vi "Thorlabs Module.vi"(7 "Actions":T3(ring)=enum."Generate Scan Pattern", 8 "error in":errorcluster, 9 "Objective":u16(ring)=1 items=["5X LKM05", "10X LKM10", "20X LKM20", "10X LSM02"], 10 "ROI Parameters":T1={"ROI (mm)"={"X (mm)"=1.0, "Y (mm)"=1.0}, "Shift (mm)"={"Xshift (mm)"=0.0, "Yshift (mm)"=0.0}}, 11 "Scan Parameters":T2={"# Scan"={"#Ascan"=400, "#Bscan"=400}, "# Rpt"={"#ARpt"=1, "#BRpt"=1}, "Aline Rate"=2, "# Extra"={"# ARpt_extra"=5, "#Brtn_extra"=60}} {"Aline Rate" items=["76 KHz", "146 KHz", "76 KHz", "28 KHz", "10 KHz"]}) -> (0 "error out":errorcluster, 2 "Data Out":sgl[][](array[numeric]), 3 "Raw Data Out":u16[][](array[numeric]))   [LabVIEW 2017]
uses:
  Program Files/Thorlabs/SpectralRadar/LabVIEW/2012/user.lib/SpectralRadar.llb/Processing Flag Selection.ctl
  Program Files/Thorlabs/SpectralRadar/LabVIEW/2012/user.lib/SpectralRadar.llb/Probe Parameter Int Selection.ctl
  Program Files/Thorlabs/SpectralRadar/LabVIEW/2012/user.lib/SpectralRadar.llb/Scan Pattern.lvclass
  Program Files/Thorlabs/SpectralRadar/LabVIEW/2012/user.lib/SpectralRadar.llb/set Spectrum Output.vi
  Program Files/Thorlabs/SpectralRadar/LabVIEW/2012/user.lib/SpectralRadar.llb/set Scan Output.vi
  Program Files/Thorlabs/SpectralRadar/LabVIEW/2012/user.lib/SpectralRadar.llb/Data.lvclass
  Program Files/Thorlabs/SpectralRadar/LabVIEW/2012/user.lib/SpectralRadar.llb/Raw Data.lvclass
  Program Files/Thorlabs/SpectralRadar/LabVIEW/2012/user.lib/SpectralRadar.llb/Processing.lvclass
  Program Files/Thorlabs/SpectralRadar/LabVIEW/2012/user.lib/SpectralRadar.llb/Probe.lvclass
  Program Files/Thorlabs/SpectralRadar/LabVIEW/2012/user.lib/SpectralRadar.llb/OCT Device.lvclass
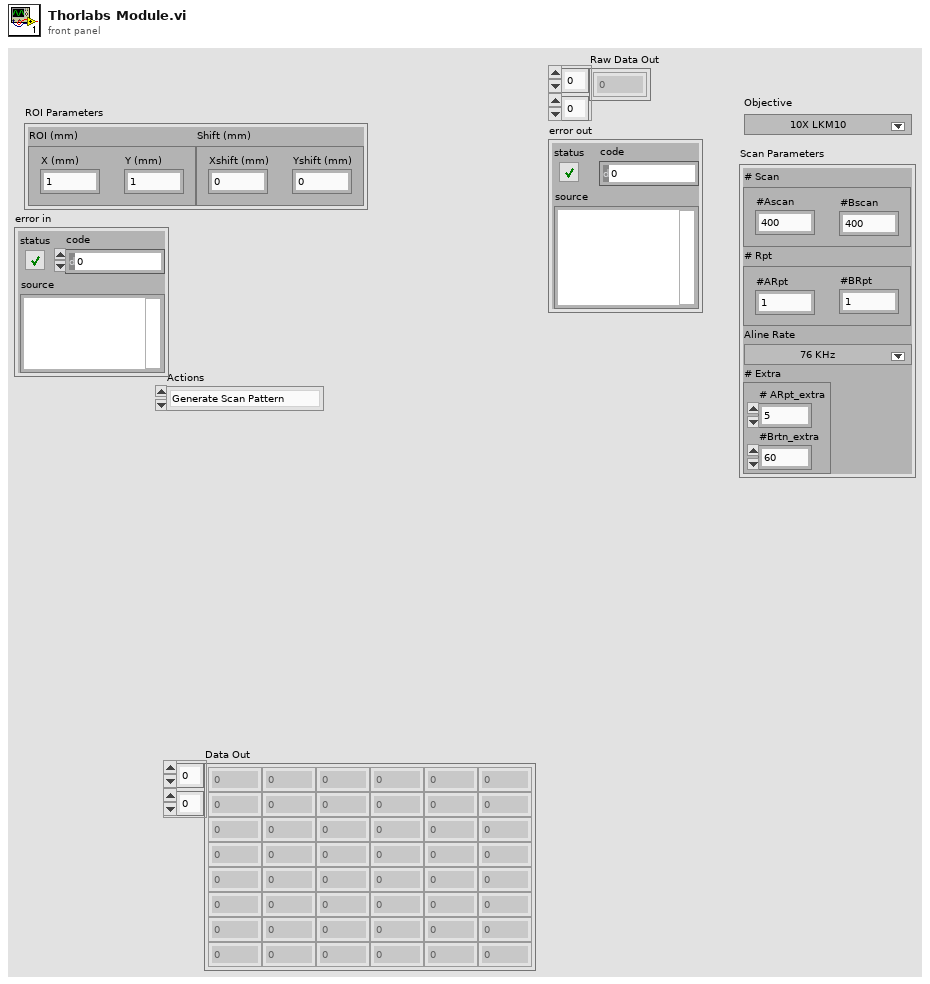
[diagram p1: front panel]
types:
  T1 = cluster{"ROI (mm)":cluster{"X (mm)":sgl, "Y (mm)":sgl}, "Shift (mm)":cluster{"Xshift (mm)":sgl, "Yshift (mm)":sgl}}
  T2 = cluster{"# Scan":cluster{"#Ascan":i32, "#Bscan":i32}, "# Rpt":cluster{"#ARpt":i32, "#BRpt":i32}, "Aline Rate":i32, "# Extra":cluster{"# ARpt_extra":i32, "#Brtn_extra":i32}}
  T3 = enum16{"Init", "Configure", "Configure Data", "Generate Scan Pattern", "Start Acquire Raw", "Start Acquire Data", "Acquire RAW", "Acquire Data", "Stop Acquire", "Uninit"}
  T4 = typedef "Processing.lvclass/Processing Flag Selection.ctl" = enum16{"Use Offset Errors", "Remove DC Spectrum", "Remove Advanced DC Spectrum", "Use Apodization", "Use Scan For Apodization", "Filter Undersampled Signals", "Use Dispersion Compensation", "Use Dechirp", "Use Extended Adjust", "Full Range Output", "Filter DC", "Autocorrelation Compensation", "DEFR", "Only Windowing", "Remove Fixed Pattern"}
  T5 = enum16{"FreeRunning", "TrigBoard_ExternalStart", "External_AScan"}
  T6 = typedef "Probe.lvclass/Probe Parameter Int Selection.ctl" = enum16{"Apodization Cycles", "Oversampling", "White Balance Auto", "Oversampling Slow Axis"}
  T7 = enum16{"Asynchronous Continuous", "Asynchronous Finite", "Synchronous"}
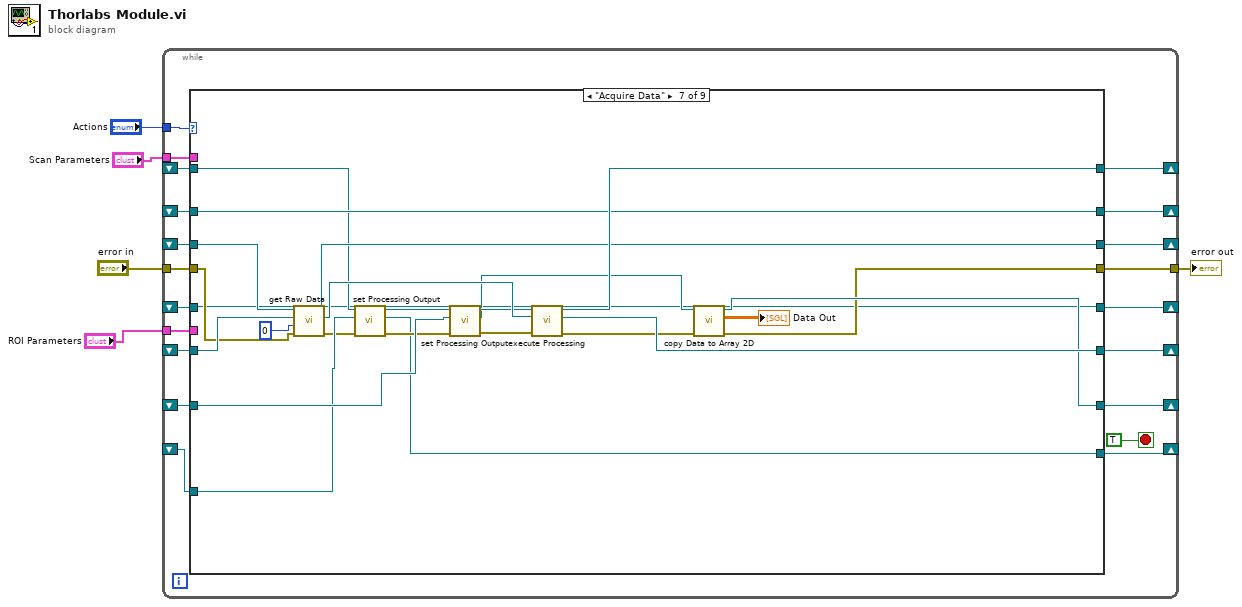
[diagram p0: block diagram]
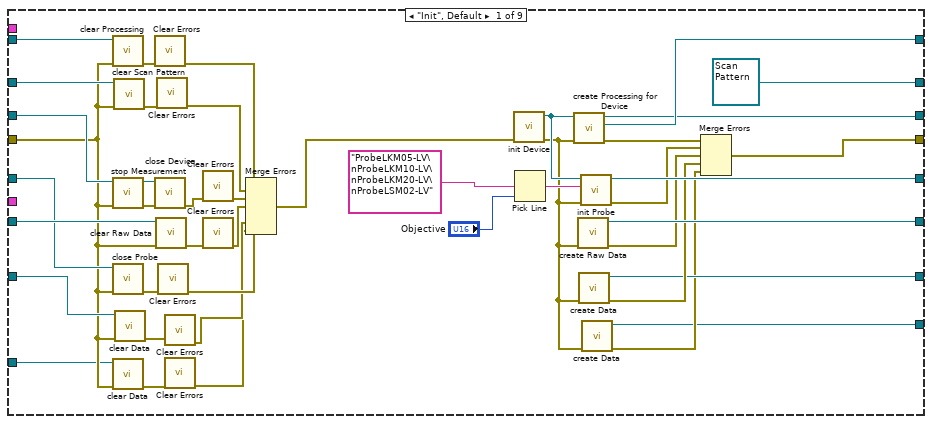
[diagram p2: hidden frame]
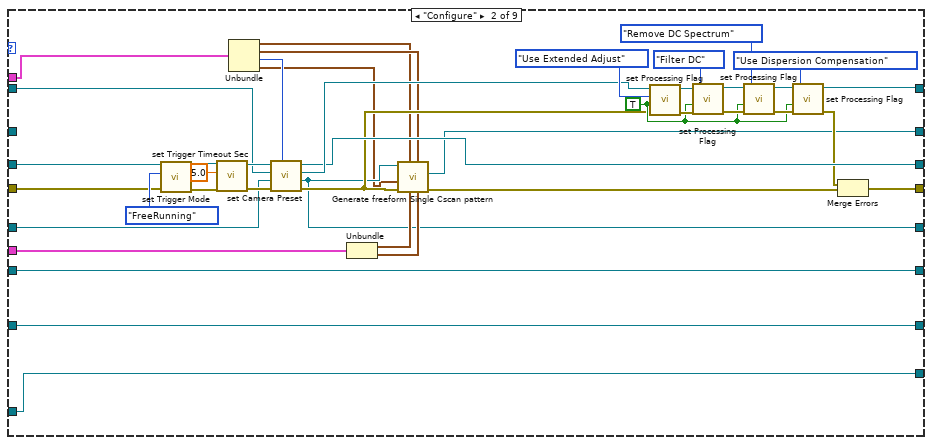
[diagram p3: hidden frame]
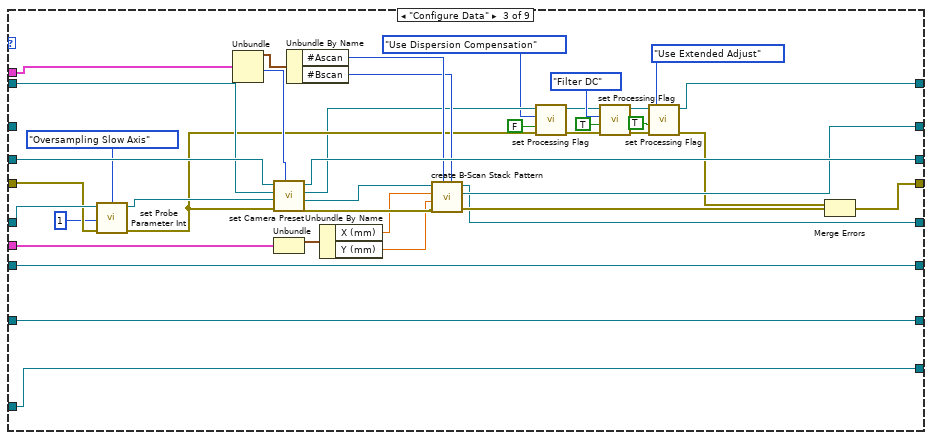
[diagram p4: hidden frame]
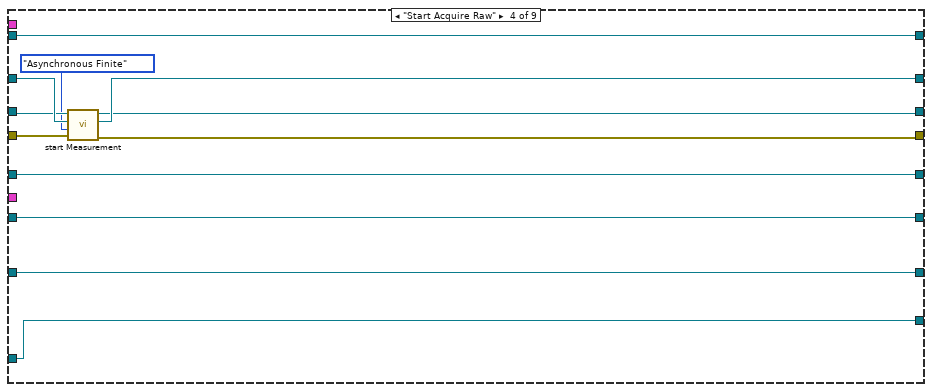
[diagram p5: hidden frame]
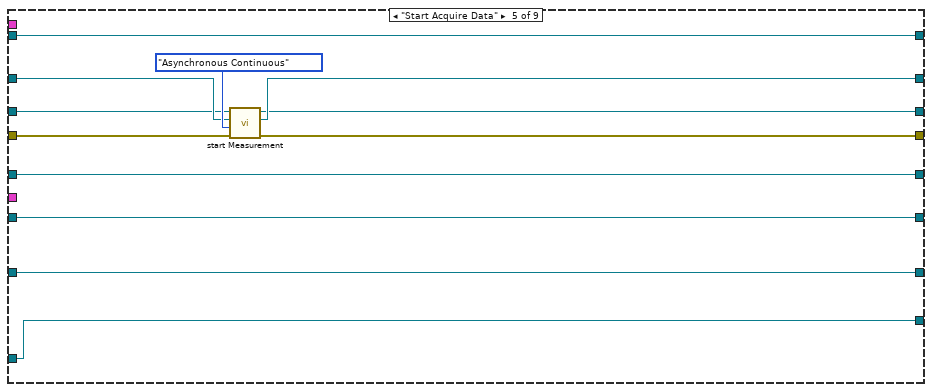
[diagram p6: hidden frame]
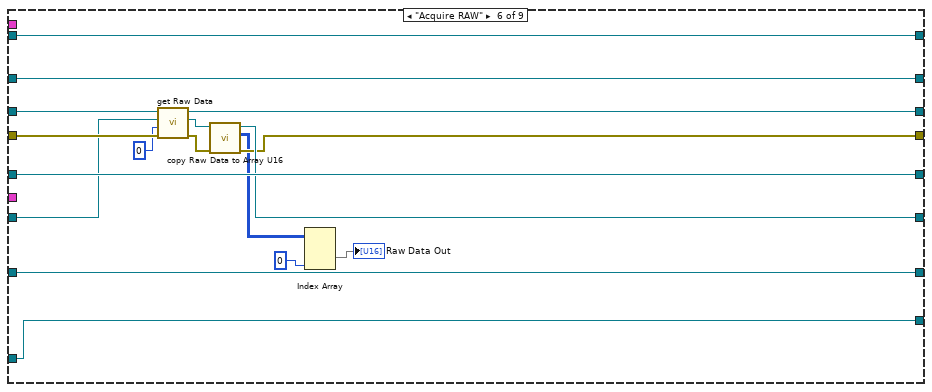
[diagram p7: hidden frame]
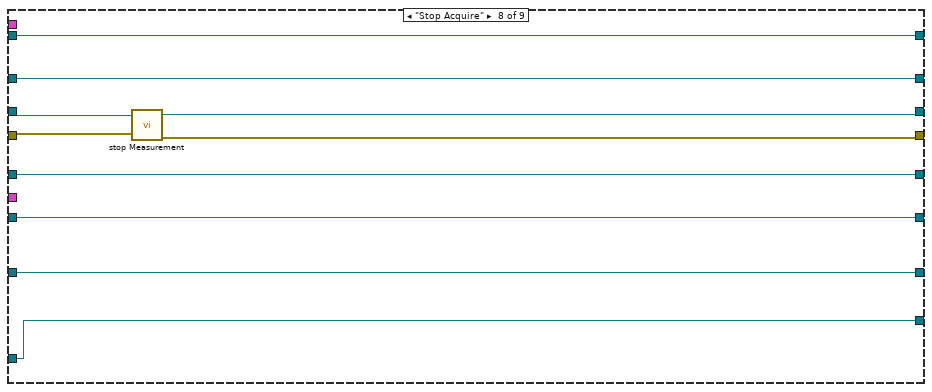
[diagram p8: hidden frame]
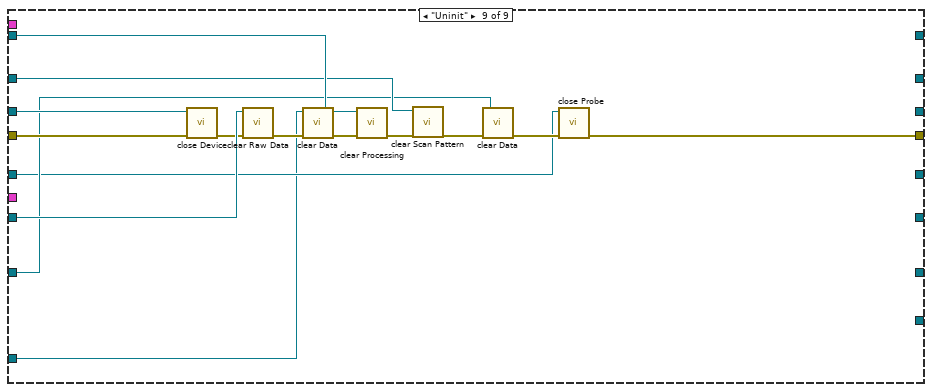
[diagram p9: hidden frame]
diagram:
  n1 = while {
    tunnel: "Actions" -> [w25]
    shift-right: [w23] -> _
    shift-left: _ -> [w19]
    shift-right: [w20] -> _
    shift-left: _ -> [w18]
    shift-right: [w17] -> _
    shift-left: _ -> [w16]
    shift-right: [w15] -> _
    shift-left: _ -> [w14]
    shift-right: [w13] -> _
    shift-left: _ -> [w12]
    tunnel: "error in" -> [w21]
    tunnel: [w22] -> w4
    shift-right: [w11] -> _
    shift-left: _ -> [w10]
    shift-right: [w9] -> _
    shift-left: _ -> [w8]
    tunnel: "Scan Parameters" -> [w7]
    tunnel: "ROI Parameters" -> [w6]
    stop <- TRUE stop-if-true
    n2 = case shown="\"Acquire Data\"" w25 {
      tunnel: [w55 w99 w145 w156 w167 w184 w207 w221 _] -> w23
      tunnel: [w61 w108 w132 w160 w171 w179 w192 w223 w229] -> w22
      tunnel: w21 -> [w30 w96 w142 w161 w172 w188 w206 w224 w233]
      tunnel: [w63 w71 w127 w154 w165 w189 w191 w218 _] -> w20
      tunnel: w19 -> [w52 w95 w146 w157 w168 w186 w213 w222 w237]
      tunnel: w18 -> [w49 w90 w144 w154 w165 w189 w191 w218 w228]
      tunnel: [w57 w83 w111 w155 w166 w190 w210 w219 _] -> w17
      tunnel: w16 -> [w47 w97 w139 w155 w166 w190 w203 w219 w236]
      tunnel: [w64 w100 w130 w153 w164 w180 w208 w217 _] -> w15
      tunnel: w14 -> [w50 w100 w130 w153 w164 w185 w214 w217 w239]
      tunnel: [refnum<class "Scan Pattern.lvclass"> refnum ("Scan Pattern") w69 w131 w158 w169 w183 w209 w220 _] -> w13
      tunnel: w12 -> [w48 _ _ w159 w170 w183 w209 w220 w234]
      tunnel: [w42 w94 w129 w151 w163 w175 w195 w216 _] -> w11
      tunnel: w10 -> [w40 w94 w129 w151 w163 w175 w205 w216 w232]
      tunnel: [w31 w93 w128 w150 w162 w174 w194 w215 _] -> w9
      tunnel: w8 -> [w27 w93 w128 w150 w162 w174 w204 w215 w225]
      tunnel: w7 -> [_ w92 w126 _ _ _ _ _ _]
      tunnel: w6 -> [_ w91 w125 _ _ _ _ _ _]
      frame "Init", Default {
        n3 = call "clear Processing.vi"("error in (no error)"=w30, "Processing"=w47) -> ("error out"=w46:errorcluster)  [unwired: 5 in]
        n4 = call "stop Measurement.vi"("error in (no error)"=w30, "OCTDevice"=w52) -> ("error out"=w54:errorcluster, "OCTDevice"=w53:refnum<class "OCT Device.lvclass">)  [unwired: 4 in]
        n5 = call "close Probe.vi"("error in (no error)"=w30, "GalvoControl"=w49) -> ("error out"=w45:errorcluster)  [unwired: 5 in]
        n6 = call "clear Data.vi"("error in (no error)"=w30, "Data"=w27) -> ("error out"=w29:errorcluster)  [unwired: 5 in]
        n7 = call "clear Scan Pattern.vi"("error in (no error)"=w30, "Scan Pattern in"=w48) -> ("error out"=w44:errorcluster)  [unwired: 5 in]
        n8 = call "clear Data.vi"("error in (no error)"=w30, "Data"=w40) -> ("error out"=w41:errorcluster)  [unwired: 5 in]
        n9 = call <vilib>:"Clear Errors.vi"("error in (no error)"=w46) -> ("error out"=w39:errorcluster)  [unwired: 5 in, 1 out]
        n10 = call "close Device.vi"("error in (no error)"=w54, "OCTDevice"=w53) -> ("error out"=w66:errorcluster)  [unwired: 5 in]
        n11 = call "clear Raw Data.vi"("error in (no error)"=w30, "Raw Data"=w50) -> ("error out"=w65:errorcluster)  [unwired: 5 in]
        n12 = call <vilib>:"Clear Errors.vi"("error in (no error)"=w44) -> ("error out"=w38:errorcluster)  [unwired: 5 in, 1 out]
        n13 = call <vilib>:"Clear Errors.vi"("error in (no error)"=w45) -> ("error out"=w35:errorcluster)  [unwired: 5 in, 1 out]
        n14 = call <vilib>:"Clear Errors.vi"("error in (no error)"=w41) -> ("error out"=w34:errorcluster)  [unwired: 5 in, 1 out]
        n15 = call <vilib>:"Clear Errors.vi"("error in (no error)"=w29) -> ("error out"=w28:errorcluster)  [unwired: 5 in, 1 out]
        n16 = call <vilib>:"Clear Errors.vi"("error in (no error)"=w66) -> ("error out"=w37:errorcluster)  [unwired: 5 in, 1 out]
        n17 = call <vilib>:"Clear Errors.vi"("error in (no error)"=w65) -> ("error out"=w36:errorcluster)  [unwired: 5 in, 1 out]
        n18 = Merge Errors(w39, w38, w37, w36, w35, w34, w28) -> (w32:errorcluster)
        n19 = call "init Device.vi"("error in (no error)"=w32) -> ("error out"=w26:errorcluster, "OCTDevice"=w58:refnum<class "OCT Device.lvclass">)  [unwired: 5 in]
        n20 = Pick Line(multi-line string="ProbeLKM05-LV\nProbeLKM10-LV\nProbeLKM20-LV\nProbeLSM02-LV" ("string (\"\")"), line index="Objective") -> (output string=w62:string)  [unwired: 1 in]
        n21 = call "create Processing for Device.vi"("error in (no error)"=w26, "OCTDevice"=w58) -> ("error out"=w56:errorcluster, "Processing"=w57:refnum<class "Processing.lvclass">, "OCTDevice"=w55:refnum<class "OCT Device.lvclass">)  [unwired: 3 in]
        n22 = call "create Raw Data.vi"("error in (no error)"=w26) -> ("error out"=w59:errorcluster, "Raw Data"=w64:refnum<class "Raw Data.lvclass">)  [unwired: 5 in]
        n23 = call "create Data.vi"("error in (no error)"=w26) -> ("error out"=w43:errorcluster, "Data"=w42:refnum<class "Data.lvclass">)  [unwired: 5 in]
        n24 = call "init Probe.vi"("error in (no error)"=w26, "Probe"=w62, "OCT Device"=w58) -> ("error out"=w60:errorcluster, "GalvoControl"=w63:refnum<class "Probe.lvclass">)  [unwired: 3 in]
        n25 = call "create Data.vi"("error in (no error)"=w26) -> ("error out"=w33:errorcluster, "Data"=w31:refnum<class "Data.lvclass">)  [unwired: 5 in]
        n26 = Merge Errors(w56, w60, w59, w43, w33) -> (w61:errorcluster)
      }
      frame "Configure" {
        w80 = TRUE ("Flag")
        n27 = call "set Trigger Mode.vi"("error in (no error)"=w96, "Trigger Type"=T5."FreeRunning", "OCTDevice in"=w95) -> ("error out"=w107:errorcluster, "OCTDevice out"=w109:refnum<class "OCT Device.lvclass">)  [unwired: 3 in]
        n28 = call "set Trigger Timeout Sec.vi"("error in (no error)"=w107, "Trigger Timeout"=5.0, "OCTDevice in"=w109) -> ("error out"=w102:errorcluster, "OCTDevice out"=w101:refnum<class "OCT Device.lvclass">)  [unwired: 3 in]
        n29 = Unbundle(w92) -> ("# Scan"=w72:cluster{"#Ascan":i32, "#Bscan":i32}, "# Rpt"=w73:cluster{"#ARpt":i32, "#BRpt":i32}, "Aline Rate"=w98:i32, "# Extra"=w70:cluster{"# ARpt_extra":i32, "#Brtn_extra":i32})
        n30 = call "set Camera Preset.vi"("Numeric"=w98, "error in (no error)"=w102, "Probe"=w90, "Processing"=w97, "OCTDevice"=w101) -> ("error out"=w77:errorcluster, "Probe 2"=w71:refnum<class "Probe.lvclass">, "Processing"=w103:refnum<class "Processing.lvclass">, "OCTDevice out"=w99:refnum<class "OCT Device.lvclass">)  [unwired: 1 in]
        n31 = Unbundle(w91) -> ("ROI (mm)"=w75:cluster{"X (mm)":sgl, "Y (mm)":sgl}, "Shift (mm)"=w74:cluster{"Xshift (mm)":sgl, "Yshift (mm)":sgl})
        n32 = call "Generate freeform Single Cscan pattern.vi"("Shift (mm)"=w74, "# Rpt"=w73, "ROI (mm)"=w75, "# Scan"=w72, "error in (no error)"=w77, "# Extra"=w70, "Probe"=w71) -> ("error out"=w76:errorcluster, "Scan Pattern"=w69:refnum<class "Scan Pattern.lvclass">)  [unwired: 1 in, 2 out]
        n33 = call "set Processing Flag.vi"("error in (no error)"=w77, "Flag"=w80, "Processing Flag Selection"=Processing_Flag_Selection."Use Extended Adjust", "Processing"=w103) -> ("error out"=w89:errorcluster, "Processing"=w88:refnum<class "Processing.lvclass">)  [unwired: 2 in]
        n34 = call "set Processing Flag.vi"("error in (no error)"=w89, "Flag"=w80, "Processing Flag Selection"=Processing_Flag_Selection."Filter DC", "Processing"=w88) -> ("error out"=w86:errorcluster, "Processing"=w82:refnum<class "Processing.lvclass">)  [unwired: 2 in]
        n35 = call "set Processing Flag.vi"("error in (no error)"=w86, "Flag"=w80, "Processing Flag Selection"=Processing_Flag_Selection."Remove DC Spectrum", "Processing"=w82) -> ("error out"=w85:errorcluster, "Processing"=w81:refnum<class "Processing.lvclass">)  [unwired: 2 in]
        n36 = call "set Processing Flag.vi"("error in (no error)"=w85, "Flag"=w80, "Processing Flag Selection"=Processing_Flag_Selection."Use Dispersion Compensation", "Processing"=w81) -> ("error out"=w84:errorcluster, "Processing"=w83:refnum<class "Processing.lvclass">)  [unwired: 2 in]
        n37 = Merge Errors(w84, w76) -> (w108:errorcluster)
      }
      frame "Configure Data" {
        n38 = call "set Probe Parameter Int.vi"("error in (no error)"=w142, "Value"=1, "Probe Parameter Int"=Probe_Parameter_Int_Selection."Oversampling Slow Axis", "GalvoControl"=w144) -> ("error out"=w124:errorcluster, "GalvoControl"=w143:refnum<class "Probe.lvclass">)  [unwired: 2 in]
        n39 = Unbundle(w126) -> ("# Scan"=w136:cluster{"#Ascan":i32, "#Bscan":i32}, "Aline Rate"=w149:i32)  [unwired: 2 out]
        n40 = call "set Camera Preset.vi"("Numeric"=w149, "error in (no error)"=w124, "Probe"=w143, "Processing"=w139, "OCTDevice"=w146) -> ("error out"=w138:errorcluster, "Probe 2"=w137:refnum<class "Probe.lvclass">, "Processing"=w118:refnum<class "Processing.lvclass">, "OCTDevice out"=w145:refnum<class "OCT Device.lvclass">)  [unwired: 1 in]
        n41 = Unbundle(w125) -> ("ROI (mm)"=w147:cluster{"X (mm)":sgl, "Y (mm)":sgl})  [unwired: 1 out]
        n42 = Unbundle By Name(w136) -> ("#Ascan"=w135:i32, "#Bscan"=w134:i32)
        n43 = Unbundle By Name(w147) -> ("X (mm)"=w123:sgl, "Y (mm)"=w122:sgl)
        n44 = call "create B-Scan Stack Pattern.vi"("Size Y"=w134, "Size X"=w135, "error in (no error)"=w138, "Range Y"=w122, "Range X"=w123, "Probe"=w137) -> ("error out"=w133:errorcluster, "Scan Pattern"=w131:refnum<class "Scan Pattern.lvclass">, "Probe"=w127:refnum<class "Probe.lvclass">)  [unwired: 1 in]
        n45 = call "set Processing Flag.vi"("error in (no error)"=w124, "Flag"=FALSE, "Processing Flag Selection"=Processing_Flag_Selection."Use Dispersion Compensation", "Processing"=w118) -> ("error out"=w119:errorcluster, "Processing"=w117:refnum<class "Processing.lvclass">)  [unwired: 2 in]
        n46 = call "set Processing Flag.vi"("error in (no error)"=w119, "Flag"=TRUE, "Processing Flag Selection"=Processing_Flag_Selection."Filter DC", "Processing"=w117) -> ("error out"=w148:errorcluster, "Processing"=w112:refnum<class "Processing.lvclass">)  [unwired: 2 in]
        n47 = call "set Processing Flag.vi"("error in (no error)"=w148, "Flag"=TRUE, "Processing Flag Selection"=Processing_Flag_Selection."Use Extended Adjust", "Processing"=w112) -> ("error out"=w114:errorcluster, "Processing"=w111:refnum<class "Processing.lvclass">)  [unwired: 2 in]
        n48 = Merge Errors(w114, w133) -> (w132:errorcluster)
      }
      frame "Start Acquire Raw" {
        n49 = call "start Measurement.vi"("error in (no error)"=w161, "Acquisition Type"=T7."Asynchronous Finite", "Scan Pattern"=w159, "OCTDevice"=w157) -> ("error out"=w160:errorcluster, "Scan Pattern"=w158:refnum<class "Scan Pattern.lvclass">, "OCTDevice"=w156:refnum<class "OCT Device.lvclass">)  [unwired: 1 in]
      }
      frame "Start Acquire Data" {
        n50 = call "start Measurement.vi"("error in (no error)"=w172, "Acquisition Type"=T7."Asynchronous Continuous", "Scan Pattern"=w170, "OCTDevice"=w168) -> ("error out"=w171:errorcluster, "Scan Pattern"=w169:refnum<class "Scan Pattern.lvclass">, "OCTDevice"=w167:refnum<class "OCT Device.lvclass">)  [unwired: 1 in]
      }
      frame "Acquire RAW" {
        n51 = call "get Raw Data.vi"("error in (no error)"=w188, "Camera Index"=0, "RawData in"=w185, "OCTDevice in"=w186) -> ("error out"=w182:errorcluster, "RawData out"=w181:refnum<class "Raw Data.lvclass">, "OCTDevice out"=w184:refnum<class "OCT Device.lvclass">)  [unwired: 1 in]
        n52 = call "copy Raw Data to Array U16.vi"("error in (no error)"=w182, "Data in"=w181) -> ("error out"=w179:errorcluster, "Data Content"=w177:u16[][][], "Data out"=w180:refnum<class "Raw Data.lvclass">)  [unwired: 3 in]
        n53 = Index Array(array=w177, index (dim 2)=0 ("index (page)")) -> (element=→"Raw Data Out":u16[][])  [unwired: 2 in]
      }
      frame "Acquire Data" {
        n54 = call "get Raw Data.vi"("error in (no error)"=w206, "Camera Index"=0, "RawData in"=w214, "OCTDevice in"=w213) -> ("error out"=w202:errorcluster, "RawData out"=w211:refnum<class "Raw Data.lvclass">, "OCTDevice out"=w207:refnum<class "OCT Device.lvclass">)  [unwired: 1 in]
        n55 = call-poly "set Processing Output.vi"("error in (no error)"=w202, "Data"=w204, "Processing"=w203) -> ("error out"=w201:errorcluster, "Data"=w194:refnum<class "Data.lvclass">, "Processing"=w199:refnum<class "Processing.lvclass">)  [unwired: 2 in]
        n56 = call-poly "set Processing Output.vi"("error in (no error)"=w201, "Data"=w205, "Processing"=w199) -> ("error out"=w212:errorcluster, "Data"=w197:refnum<class "Data.lvclass">, "Processing"=w198:refnum<class "Processing.lvclass">)  [unwired: 2 in]
        n57 = call "execute Processing.vi"("error in (no error)"=w212, "Raw Data"=w211, "Processing"=w198) -> ("error out"=w193:errorcluster, "Raw Data"=w208:refnum<class "Raw Data.lvclass">, "Processing"=w210:refnum<class "Processing.lvclass">)  [unwired: 2 in]
        n58 = call "copy Data to Array 2D.vi"("error in (no error)"=w193, "Data in"=w197) -> ("error out"=w192:errorcluster, "Data Content"=→"Data Out":sgl[][], "Data out"=w195:refnum<class "Data.lvclass">)  [unwired: 3 in]
      }
      frame "Stop Acquire" {
        n59 = call "stop Measurement.vi"("error in (no error)"=w224, "OCTDevice"=w222) -> ("error out"=w223:errorcluster, "OCTDevice"=w221:refnum<class "OCT Device.lvclass">)  [unwired: 4 in]
      }
      frame "Uninit" {
        n60 = call "close Device.vi"("error in (no error)"=w233, "OCTDevice"=w237) -> ("error out"=w238:errorcluster)  [unwired: 5 in]
        n61 = call "clear Raw Data.vi"("error in (no error)"=w238, "Raw Data"=w239) -> ("error out"=w227:errorcluster)  [unwired: 5 in]
        n62 = call "clear Data.vi"("error in (no error)"=w227, "Data"=w225) -> ("error out"=w226:errorcluster)  [unwired: 5 in]
        n63 = call "clear Processing.vi"("error in (no error)"=w226, "Processing"=w236) -> ("error out"=w235:errorcluster)  [unwired: 5 in]
        n64 = call "clear Scan Pattern.vi"("error in (no error)"=w235, "Scan Pattern in"=w234) -> ("error out"=w231:errorcluster)  [unwired: 5 in]
        n65 = call "clear Data.vi"("error in (no error)"=w231, "Data"=w232) -> ("error out"=w230:errorcluster)  [unwired: 5 in]
        n66 = call "close Probe.vi"("error in (no error)"=w230, "GalvoControl"=w228) -> ("error out"=w229:errorcluster)  [unwired: 5 in]
      }
    }
  }
  "error out" <- w4
